vi "RT Driver VI.vi"(7 "Operation":T1, 11 "Device Reference in":T2 format="%.0x") -> (0 "Error Code":i32)   [LabVIEW 2016, in "LIN Frame Protection Addon Engine.lvlib"]
uses:
  LIN Frame Protection Addon Engine.lvlib
  <vilib>/NI Veristand/Custom Device API/Custom Device Item Ref.ctl
  <vilib>/NI Veristand/Custom Device API/Model Interface Driver VI Operation.ctl
  Types/RT Engine State Variables.ctl
  Types/RT Engine Generate References.ctl
  Shared/Types/FrameConfiguration.ctl
  Shared/Types/InputChannelConfiguration.ctl
  Shared/Types/Protection Type.ctl
  <vilib>/NI Veristand/Custom Device API/Block Data Reference.ctl
  <vilib>/NI Veristand/Custom Device API/Data Reference.ctl
  Types/RT Engine Monitor References.ctl
  <vilib>/NI Veristand/Custom Device API/Custom Device API.lvlib
  <vilib>/NI VeriStand/Custom Device Tools/Custom Device Utility Library/Custom Device Utility Library.lvlib
  Shared/LIN Frame Protection Addon Shared.lvlib
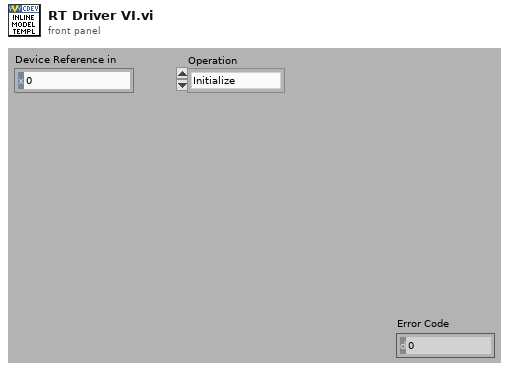
[diagram p1: front panel]
types:
  T1 = typedef "Custom Device API.lvlib/Model Interface Driver VI Operation.ctl" = enum16{"Initialize", "Start", "Execute Model", "Close"}
  T2 = typedef "Custom Device API.lvlib/Custom Device Item Ref.ctl" = u64
  T3 = typedef "LIN Frame Protection Addon Engine.lvlib/RT Engine State Variables.ctl" = cluster{"Generate Frame Configurations":T4[], "PCL Rate (secs)":dbl, "Monitor Frame Configurations":T10[]}
  T4 = typedef "LIN Frame Protection Addon Engine.lvlib/RT Engine Generate References.ctl" = cluster{"Frame Configuration":T5, "Input Channels Values":dbl[], "Input Channels Refs":T8[], "CD Results Values":dbl[], "CD Results Refs":T8[], "Conversion":refnum<k21>}
  T5 = typedef "LIN Frame Protection Addon Shared.lvlib/FrameConfiguration.ctl" = cluster{"Input Channels":T6[], "Schedule_SumOfDelays":dbl, "Rolling Counter Count":dbl, "PCL Count":u64, "Max Count":dbl, "Frame ID":u32, "Rolling Counter":T6, "CRC":T6, "Frame Name":string, "Cluster":string, "Database":string, "Protection Type":T7}
  T6 = typedef "LIN Frame Protection Addon Shared.lvlib/InputChannelConfiguration.ctl" = cluster{"Start Bit":i32, "Name":string, "Node Path":string, "Number of bits":i32, "Scale":dbl, "Offset":dbl, "Data Type":u32}
  T7 = typedef "LIN Frame Protection Addon Shared.lvlib/Protection Type.ctl" = enum16{"Checksum", "CRC", "None (Counter Only)"}
  T8 = typedef "Custom Device API.lvlib/Block Data Reference.ctl" = cluster{"Data Reference":T9, "Offset":u64, "Length":u64}
  T9 = typedef "Custom Device API.lvlib/Data Reference.ctl" = i32
  T10 = typedef "LIN Frame Protection Addon Engine.lvlib/RT Engine Monitor References.ctl" = cluster{"Frame Configuration":T5, "Input Channels Values":dbl[], "Input Channels Refs":T8[], "CD Results Values":dbl[], "CD Results Refs":T8[], "Validation Channels Values":dbl[], "Validation Channels Refs":T8[], "Conversion":refnum<k21>}
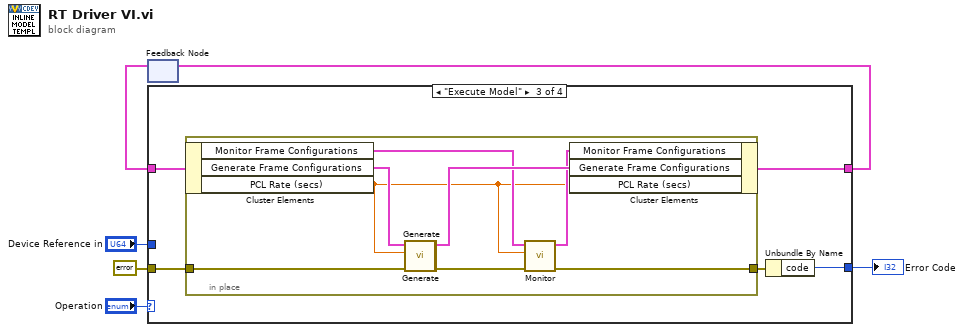
[diagram p0: block diagram]
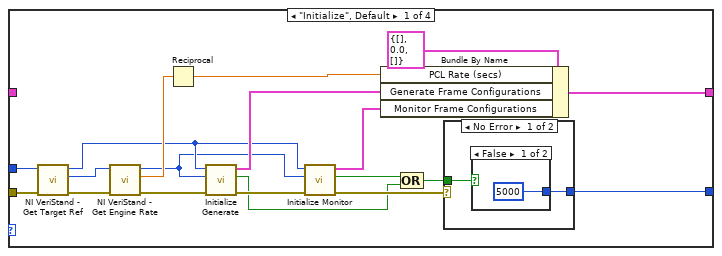
[diagram p2: hidden frame]
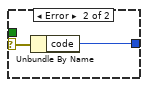
[diagram p4: hidden frame]
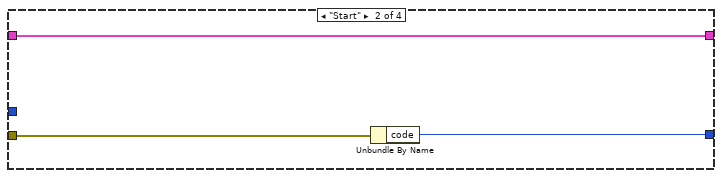
[diagram p5: hidden frame]
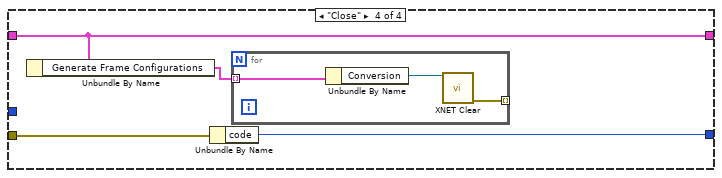
[diagram p6: hidden frame]
diagram:
  n1 = feedback #1() -> (w4:T3)  [unwired: 1 out]
  n2 = case shown="\"Execute Model\"" "Operation" {
    tunnel: [w22 w33 w34 w48] -> w5
    tunnel: w4 -> [_ w33 w35 w48]
    tunnel: "Device Reference in" -> [w17 _ _ _]
    tunnel: [w25 w31 w38 w50] -> w2
    tunnel: errorcluster {"status"=FALSE, "code"=0, "source"=""} ("error in (no error)") -> [w19 w32 w37 w49]
    frame "Initialize", Default {
      n3 = call <vilib>:"NI VeriStand - Get Target Ref.vi"("error in"=w19, "Item Ref in"=w17) -> ("error out"=w20:errorcluster, "Target Ref"=w21:T2, "Item Ref out"=w8:T2)  [unwired: 6 in, 1 out]
      n4 = call <vilib>:"NI VeriStand - Get Engine Rate.vi"("error in (no error)"=w20, "Item Ref in"=w21) -> ("error out"=w18:errorcluster, "Rate (Hz)"=w16:dbl, "Item Ref out"=w7:T2)  [unwired: 7 in]
      n5 = Reciprocal(x=w16) -> (1/x=w15:dbl)
      n6 = call "Initialize Generate.vi"("error in (no error)"=w18, "Target Ref in"=w7, "Addon Ref in"=w8) -> ("error out"=w14:errorcluster, "Found?"=w10:bool, "Generate Frame Configurations"=w24:T4[])  [unwired: 6 in]
      n7 = call "Initialize Monitor.vi"("error in (no error)"=w14, "Target Ref in"=w7, "Addon Ref in"=w8) -> ("error out"=w13:errorcluster, "Found?"=w11:bool, "Monitor Frame Configurations"=w12:T10[])  [unwired: 6 in]
      n8 = Bundle By Name(cluster=T3 {"Generate Frame Configurations"=[], "PCL Rate (secs)"=0.0, "Monitor Frame Configurations"=[]}, "PCL Rate (secs)"=w15, "Generate Frame Configurations"=w24, "Monitor Frame Configurations"=w12) -> (w22:T3)
      n9 = Compound Arithmetic op=OR(w11, w10) -> (w9:bool)
      n10 = case shown="No Error" w13 {
        selector: w13 -> [_ w29]
        tunnel: [w26 w30] -> w25
        tunnel: w9 -> [w27 _]
        frame No Error {
          n11 = case shown="False" w27 {
            tunnel: [5000 _] -> w26
            frame False {
            }
            frame True {
            }
          }
        }
        frame Error {
          n12 = Unbundle By Name(w29) -> ("code"=w30:i32)
        }
      }
    }
    frame "Start" {
      n13 = Unbundle By Name(w32) -> ("code"=w31:i32)
    }
    frame "Execute Model" {
      n14 = in-place {
        in-place-border: w37 -> [w46]
        in-place-border: [w42] -> w36
        n15 = in-place-cluster #2(w35) -> ("Monitor Frame Configurations"=w41:T10[], "Generate Frame Configurations"=w45:T4[], "PCL Rate (secs)"=w39:dbl)
        n16 = call "Generate.vi"("error in (no error)"=w46, "PCL Rate (secs)"=w39, "Frame Configurations"=w45) -> ("error out"=w43:errorcluster, "Frame Configurations"=w44:T4[])  [unwired: 7 in]
        n17 = call "Generate.vi"() -> ()  [unwired: 10 in, 2 out]
        n18 = call "Monitor.vi"("error in (no error)"=w43, "PCL Rate (secs)"=w39, "Frame Configurations"=w41) -> ("error out"=w42:errorcluster, "Frame Configurations"=w40:T10[])  [unwired: 7 in]
        n19 = in-place-cluster #2("Monitor Frame Configurations"=w40, "Generate Frame Configurations"=w44, "PCL Rate (secs)"=w39) -> (w34:T3)
      }
      n20 = Unbundle By Name(w36) -> ("code"=w38:i32)
    }
    frame "Close" {
      n21 = Unbundle By Name(w48) -> ("Generate Frame Configurations"=w47:T4[])
      n22 = Unbundle By Name(w49) -> ("code"=w50:i32)
      n23 = for {
        tunnel: w47 -> [w53] mode=indexing
        tunnel: [w51] -> _ mode=indexing
        n24 = Unbundle By Name(w53) -> ("Conversion"=w52:refnum<k21>)
        n25 = call <vilib>:"XNET Clear.vi"("session in"=w52) -> ("error out"=w51:errorcluster)  [unwired: 14 in]
      }
    }
  }
  "Error Code" <- w2
  n26 = feedback-in #1(w5) -> ()
